vi "Write setpoint.vi"(8 "error in (no error)":errorcluster, 10 "setpoint":sgl, 11 "SetSpectTempSetpoint in":refnum<class "SetSpectTempSetpoint.lvclass">) -> (0 "error out":errorcluster, 3 "SetSpectTempSetpoint out":refnum<class "SetSpectTempSetpoint.lvclass">)   [LabVIEW 2016, in "Commands.lvlib" / "SetSpectTempSetpoint.lvclass"]
uses:
  SetSpectTempSetpoint.lvclass
  SetSpectTempSetpoint.lvclass/SetSpectTempSetpoint.ctl
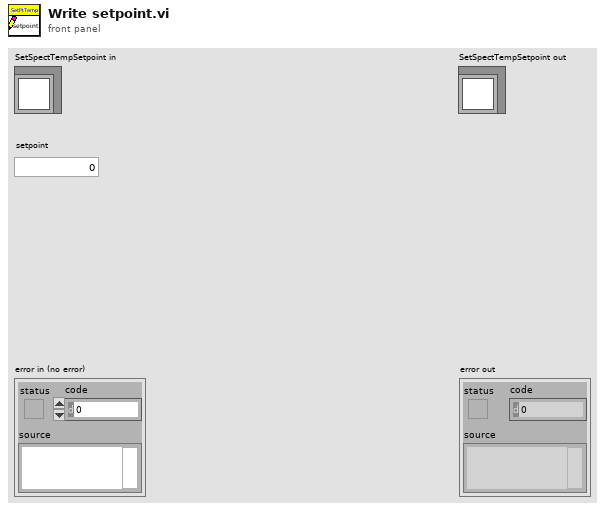
[diagram p1: front panel]
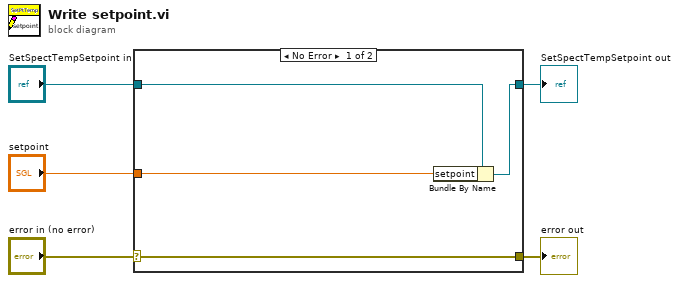
[diagram p0: block diagram]
diagram:
  n1 = case shown="No Error" "error in (no error)" {
    selector: "error in (no error)" -> [w9 w10]
    tunnel: [w9 w10] -> w4
    tunnel: [w7 w11] -> w2
    tunnel: "SetSpectTempSetpoint in" -> [w8 w11]
    tunnel: "setpoint" -> [w6 _]
    frame No Error {
      n2 = Bundle By Name(cluster=w8, "setpoint"=w6) -> (w7:refnum<class "SetSpectTempSetpoint.lvclass">)
    }
    frame Error {
    }
  }
  "error out" <- w4
  "SetSpectTempSetpoint out" <- w2
